vi "capture image.vi"() -> ()   [LabVIEW 2011]
uses:
  <vilib>/vision/driver/IMAQdx.llb/IMAQdx Camera Control Mode.ctl
  <vilib>/userdefined/High Color/IMAQdx.ctl
  <vilib>/vision/driver/NI_Vision_Acquisition_Software.lvlib
panel:
  out "fringe pattern":T1(plugin-control)
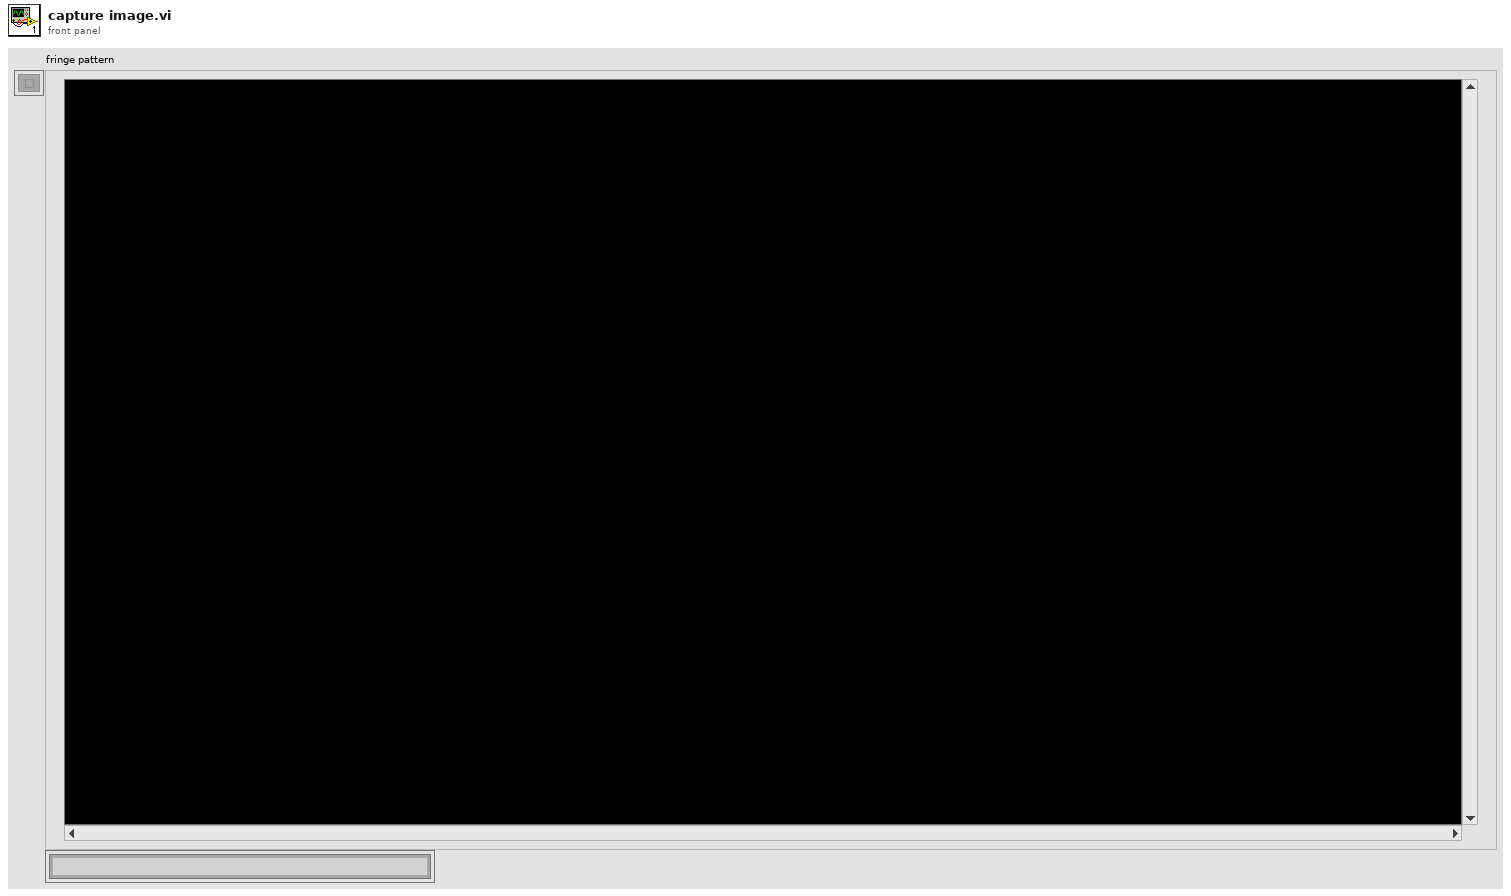
[diagram p1: front panel]
types:
  T1 = typedef "IMAQ Image.ctl" = refnum<image>
  T2 = typedef "Image Type" = u32
  T3 = typedef "IMAQdx.ctl" = refnum<k21>
  T4 = typedef "NI_Vision_Acquisition_Software.lvlib/IMAQdx Camera Control Mode.ctl" = enum32{"Controller", "Listener"}
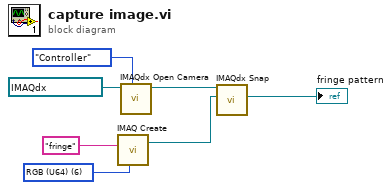
[diagram p0: block diagram]
diagram:
  w3 = T2 6 items=["Grayscale (U8)", "Grayscale (I16)", "Grayscale (SGL)", "Complex (CSG)", "RGB (U32)", "HSL (U32)", "RGB (U64)", "Grayscale (U16)"] ("Image Type")
  n1 = call "IMAQ Create"("Image Name"="fringe", "Image Type"=w3) -> ("New Image"=w1:T1)  [unwired: 2 in, 2 out]
  n2 = call <vilib>:"IMAQdx Open Camera.vi"("Camera Control Mode"=IMAQdx_Camera_Control_Mode."Controller", "Session In"=T3 "HP Webcam") -> ("Session Out"=w5:T3)  [unwired: 8 in, 1 out]
  n3 = call <vilib>:"IMAQdx Snap.vi"("Image In"=w1, "Session In"=w5) -> ("Image Out"=→"fringe pattern":T1)  [unwired: 7 in, 2 out]
